vi "Rework_Calculate.vi"(9 "Rework站号":string, 10 "当前站号":string) -> (1 "Data":string[](array[string]), 2 "Rework_List":string[](array[string]), 3 "跨站":bool)   [LabVIEW 2018]
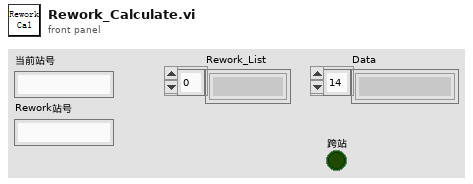
[diagram p1: front panel]
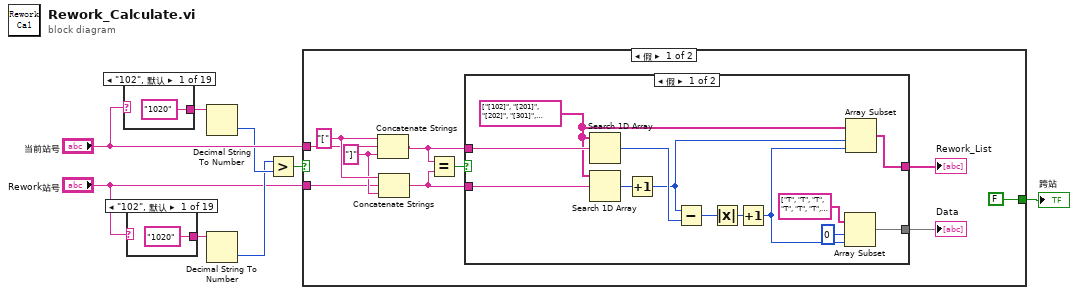
[diagram p0: block diagram]
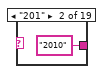
[diagram p2: hidden frame]
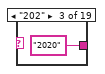
[diagram p3: hidden frame]
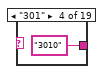
[diagram p4: hidden frame]
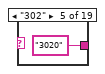
[diagram p5: hidden frame]
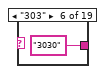
[diagram p6: hidden frame]
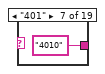
[diagram p7: hidden frame]
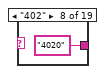
[diagram p8: hidden frame]
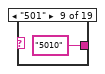
[diagram p9: hidden frame]
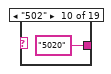
[diagram p10: hidden frame]
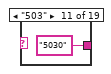
[diagram p11: hidden frame]
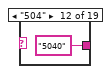
[diagram p12: hidden frame]
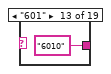
[diagram p13: hidden frame]
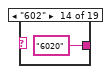
[diagram p14: hidden frame]
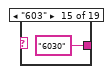
[diagram p15: hidden frame]
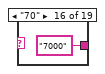
[diagram p16: hidden frame]
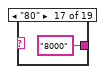
[diagram p17: hidden frame]
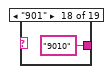
[diagram p18: hidden frame]
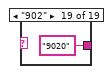
[diagram p19: hidden frame]
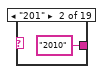
[diagram p20: hidden frame]
diagram:
  n1 = case shown="\"102\", 默认" "当前站号" {
    tunnel: ["1020" "2010" "2020" "3010" "3020" "3030" "4010" "4020" "5010" "5020" "5030" "5040" "6010" "6020" "6030" "7000" "8000" "9010" "9020"] -> w6
    frame "102", Default {
    }
    frame "201" {
    }
    frame "202" {
    }
    frame "301" {
    }
    frame "302" {
    }
    frame "303" {
    }
    frame "401" {
    }
    frame "402" {
    }
    frame "501" {
    }
    frame "502" {
    }
    frame "503" {
    }
    frame "504" {
    }
    frame "601" {
    }
    frame "602" {
    }
    frame "603" {
    }
    frame "70" {
    }
    frame "80" {
    }
    frame "901" {
    }
    frame "902" {
    }
  }
  n2 = case shown="\"102\", 默认" "Rework站号" {
    tunnel: ["1020" "2010" "2020" "3010" "3020" "3030" "4010" "4020" "5010" "5020" "5030" "5040" "6010" "6020" "6030" "7000" "8000" "9010" "9020"] -> w1
    frame "102", Default {
    }
    frame "201" {
    }
    frame "202" {
    }
    frame "301" {
    }
    frame "302" {
    }
    frame "303" {
    }
    frame "401" {
    }
    frame "402" {
    }
    frame "501" {
    }
    frame "502" {
    }
    frame "503" {
    }
    frame "504" {
    }
    frame "601" {
    }
    frame "602" {
    }
    frame "603" {
    }
    frame "70" {
    }
    frame "80" {
    }
    frame "901" {
    }
    frame "902" {
    }
  }
  n3 = Decimal String To Number(string=w6) -> (number=w5:i32)  [unwired: 2 in, 1 out]
  n4 = Decimal String To Number(string=w1) -> (number=w4:i32)  [unwired: 2 in, 1 out]
  n5 = Greater?(x=w4, y=w5) -> (0:w3:bool)
  n6 = case shown="假" w3 {
    tunnel: "当前站号" -> [w49 _]
    tunnel: "Rework站号" -> [w48 _]
    tunnel: [FALSE TRUE] -> w8
    frame False {
      w50 = "]" ("字符串")
      w51 = "[" ("字符串")
      n7 = Concatenate Strings(w51, w49, w50) -> (w53:string)
      n8 = Concatenate Strings(w51, w48, w50) -> (w52:string)
      n9 = Equal?(x=w53, y=w52) -> (x = y?=w56:bool)
      n10 = case shown="假" w56 {
        tunnel: w52 -> [w68 w74]
        tunnel: [w65 w71] -> w55
        tunnel: [w58 string[] ["T"]] -> w54
        tunnel: w53 -> [w69 _]
        frame False {
          w57 = string[] ["[102]", "[201]", "[202]", "[301]", "[302]", "[303]", "[401]", "[402]", "[501]", "[502]", "[503]", "[504]", "[601]", "[602]", "[603]", "[70]", "[80]", "[901]", "[902]"]
          n11 = Search 1D Array(1D array=w57, element=w69) -> (index of element=w67:i32)  [unwired: 1 in]
          n12 = Search 1D Array(1D array=w57, element=w68) -> (index of element=w61:i32)  [unwired: 1 in]
          n13 = Increment(x=w61) -> (x+1=w60:i32)
          n14 = Subtract(x=w60, y=w67) -> (x-y=w66:i32)
          n15 = Absolute Value(x=w66) -> (abs(x)=w63:i32)
          n16 = Increment(x=w63) -> (x+1=w62:i32)
          n17 = Array Subset(array=string[] ["T", "T", "T", "T", "T", "T", "T", "T", "T", "T", "T", "T", "T", "T", "T", "T", "T", "T", "T", "T", "T", "T", "T", "T", "T", "T"], index=0 ("索引"), length=w62) -> (w58:string[])
          n18 = Array Subset(array=w57, index=w60, length=w62) -> (w65:string[])
        }
        frame True {
          n19 = Insert Into Array(array=string[] [] ("数组"), index=0 ("索引"), new element=w74) -> (w71:string[])
        }
      }
      "Rework_List" <- w55
      "Data" <- w54
    }
    frame True {
    }
  }
  "跨站" <- w8
